vi "ts_tree_set_headers.vi"(8 "error in (no error)":errorcluster, 10 "headers":string[](array[string]), 11 "Tree.in":refnum<vi>) -> (0 "error out":errorcluster, 3 "Tree.out":refnum<vi>)   [LabVIEW 2015]
doc: "sets column headers for a tree control"
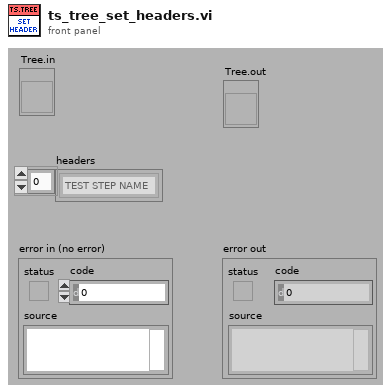
[diagram p1: front panel]
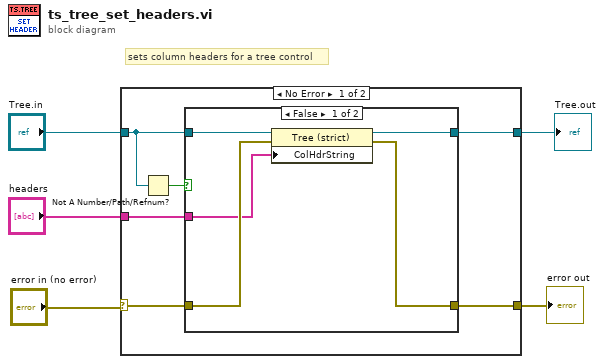
[diagram p0: block diagram]
diagram:
  # "sets column headers for a tree control"
  n1 = case shown="No Error" "error in (no error)" {
    selector: "error in (no error)" -> [w10 w19]
    tunnel: "Tree.in" -> [w6 w20]
    tunnel: [w11 w20] -> w3
    tunnel: [w9 w19] -> w2
    tunnel: "headers" -> [w8 _]
    frame No Error {
      n2 = Not A Number/Path/Refnum?(number/path/refnum=w6) -> (NaN/Path/Refnum?=w7:bool)
      n3 = case shown="False" w7 {
        tunnel: w6 -> [w16 w18]
        tunnel: [w15 w18] -> w11
        tunnel: w10 -> [w14 w17]
        tunnel: [w13 w17] -> w9
        tunnel: w8 -> [w12 _]
        frame False {
          n4 = property class="Tree (strict)"(reference=w16, error in=w14, "ColHdrString"=w12) -> (reference out=w15:refnum<vi>, error out=w13:errorcluster)
        }
        frame True {
        }
      }
    }
    frame Error {
    }
  }
  "Tree.out" <- w3
  "error out" <- w2
